vi "GoalKickKeeperTacticVSS.vi"(7 "First call?":bool=TRUE, 8 "error in (no error)":errorcluster, 9 "Game in":refnum<class "Game.lvclass">, 10 "Robot":refnum<class "Robot.lvclass">, 11 "GoalKickKeeperTacticVSS in":refnum<class "GoalKickKeeperTacticVSS.lvclass">) -> (0 "error out":errorcluster, 2 "Robot out":refnum<class "Robot.lvclass">, 3 "GoalKickKeeperTacticVSS out":refnum<class "GoalKickKeeperTacticVSS.lvclass">, 5 "x .or. y?":bool)   [LabVIEW 2020, in "GoalKickKeeperTacticVSS.lvclass"]
uses:
  GoalKickKeeperTacticVSS.lvclass
  C:/Users/pedro/Desktop/SSL_AI/Tactic_class/Tactic.lvclass
  Robot_class/Robot.lvclass
  Game_class/Game.lvclass
  Robot_class/tactics.ctl
  Tactic_class/Tactic.lvclass/Tactic.ctl
  Game_class/Game.lvclass/Game.ctl
  Robot_class/Robot.lvclass/Robot.ctl
  Game_class/Read BallRef.vi
  Tactic_class/Read Skillbook.vi
  Robot_class/Write tactic.vi
  Skillbook_class/Skillbook.lvclass
  KickSkillVSS_class/KickSkillVSS.lvclass
  PenaltyPosSkillVSS_class/PenaltyPosSkillVSS.lvclass
  BallDispPosSkillVSS_class/BallDispPosSkillVSS.lvclass
  BallToGoalSkillVSS_class/BallToGoalSkillVSS.lvclass
  GoToBallSkillVSS_class/GoToBallSkillVSS.lvclass
  DefBallPosSkillVSS_class/DefBallPosSkillVSS.lvclass
  HaltSkill_class/HaltSkill.lvclass
  KeeperDefPosSkillVSS_class/KeeperDefPosSkillVSS.lvclass
  GoToBallKeeperSkillVSS_class/GoToBallKeeperSkillVSS.lvclass
  Ball_class/Ball.lvclass
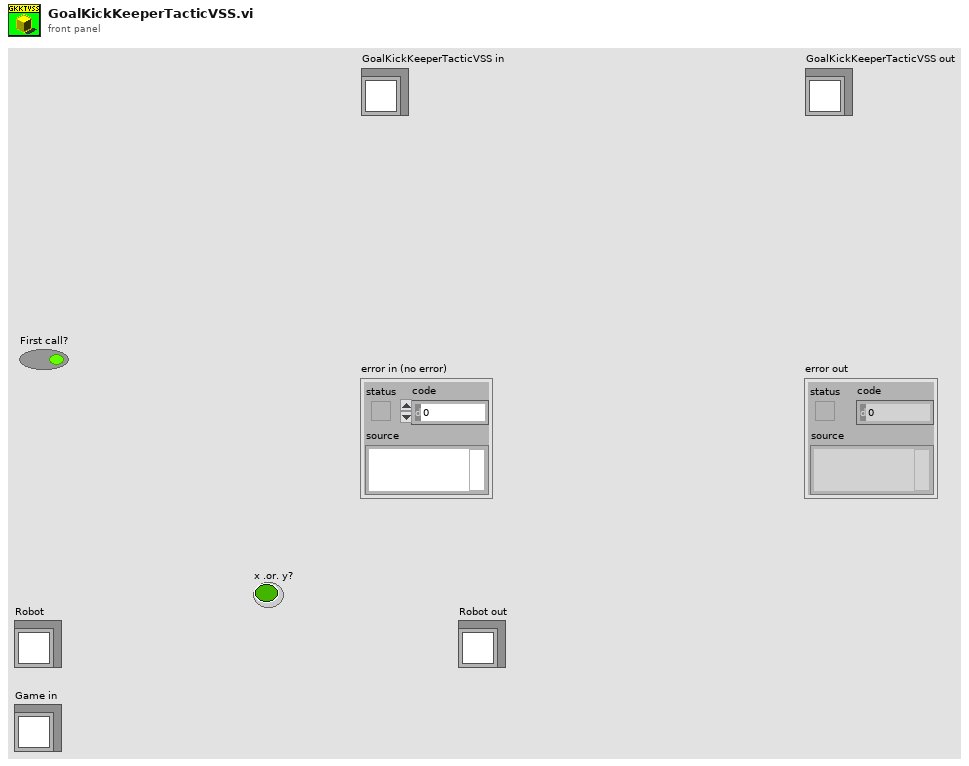
[diagram p1: front panel]
types:
  T1 = typedef "tactics.ctl" = enum16{"ReceivePassInFuturePoint", "Roller", "PrepareRollToPassRollerGoTo", "PrepareRollToPassReceiverGoTo", "WaitRoll", "PositionToRoll", "PenaltyAttacker", "PassObserver", "PenaltyDefense", "TableReceiverTactic", "Test", "DefendGoal", "Marker", "FollowAttacker", "DefendArea", "Shoot", "AttackerAimGoal", "AttackerBallOutOfField", "AttackerBlock", "AttackerStop", "Duelist", "Halt", "ZigZag", "GoTo", "Timeout", "KickToPassReceiver", "PositionToReceivePass", "DefendAreaVSS", "DefendGoalVSS", "KickVSS", "AttackVSS", "DispBallVSS", "PenaltyAttackVSS", "WaitPass"}
  T2 = cluster{"KickSkillVSS":refnum<class "KickSkillVSS.lvclass">, "PenaltyPosSkillVSS":refnum<class "PenaltyPosSkillVSS.lvclass">, "BallDispPosSkillVSS":refnum<class "BallDispPosSkillVSS.lvclass">, "BallToGoalSkillVSS":refnum<class "BallToGoalSkillVSS.lvclass">, "GoToBallSkillVSS":refnum<class "GoToBallSkillVSS.lvclass">, "DefBallPosSkillVSS":refnum<class "DefBallPosSkillVSS.lvclass">, "HaltSkill":refnum<class "HaltSkill.lvclass">, "KeeperDefPosSkillVSS":refnum<class "KeeperDefPosSkillVSS.lvclass">, "GoToBallKeeperSkillVSS":refnum<class "GoToBallKeeperSkillVSS.lvclass">}
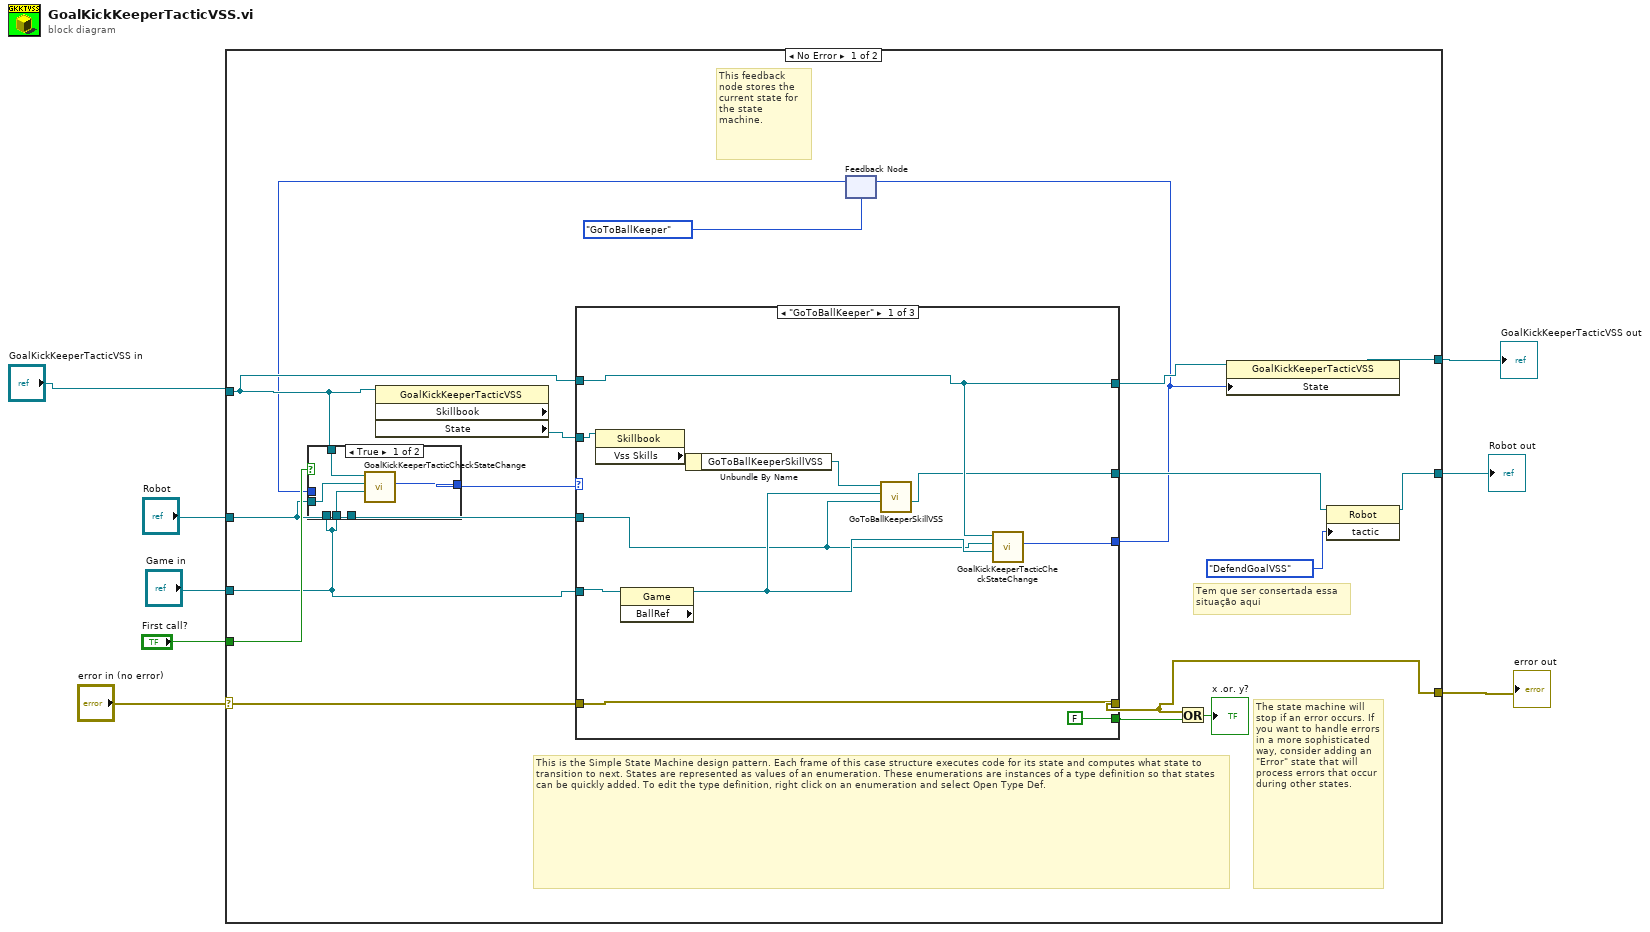
[diagram p0: block diagram]
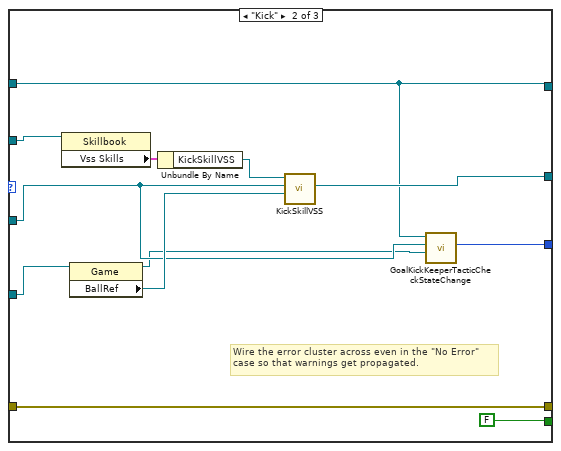
[diagram p2: hidden frame]
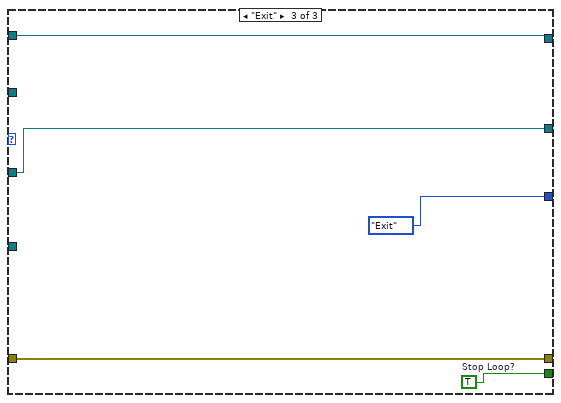
[diagram p3: hidden frame]
diagram:
  n1 = case shown="No Error" "error in (no error)" {
    selector: "error in (no error)" -> [w16 w62]
    tunnel: [w17 w62] -> w2
    tunnel: [w26 w61] -> w1
    tunnel: "GoalKickKeeperTacticVSS in" -> [w20 w61]
    tunnel: "Robot" -> [w12 w60]
    tunnel: "Game in" -> [w11 _]
    tunnel: [w24 w60] -> w5
    tunnel: "First call?" -> [w23 _]
    frame No Error {
      # "Tem que ser consertada essa \nsituação aqui"
      # "The state machine will stop if an error occurs. If you want to handle errors in a more sophisticated way, consider adding an \"Error\" state that will process errors that occur during other states."
      # "This feedback node stores the current state for the state machine."
      # "This is the Simple State Machine design pattern. Each frame of this case structure executes code for its state and computes what state to transition to next. States are represented as values of an enumeration. These enumerations are instances of a type definition so that states can be quickly added. To edit the type definition, right click on an enumeration and select Open Type Def."
      n2 = property class="GoalKickKeeperTacticVSS" props=["Skillbook", "State"](reference=w20) -> ("Skillbook"=w15:refnum<class "Skillbook.lvclass">)  [unwired: 1 in, 3 out]
      n3 = feedback #1(enum16{"GoToBallKeeper", "Kick", "Exit"}."GoToBallKeeper" ("State")) -> (w13:enum16{"GoToBallKeeper", "Kick", "Exit"})
      n4 = case shown="True" w23 {
        tunnel: w20 -> [w55 _]
        tunnel: w12 -> [_ _]
        tunnel: w11 -> [w58 _]
        tunnel: [w56 w59] -> w14
        tunnel: w13 -> [_ w59]
        tunnel: w12 -> [w57 _]
        tunnel: w11 -> [_ _]
        frame True {
          n5 = call "GoalKickKeeperTacticCheckStateChange.vi"("Game in"=w58, "Robot In"=w57, "GoalKickKeeperTacticVSS in"=w55) -> ("States"=w56:enum16{"GoToBallKeeper", "Kick", "Exit"})  [unwired: 6 in, 2 out]
        }
        frame False {
        }
      }
      n6 = case shown="\"GoToBallKeeper\"" w14 {
        tunnel: w11 -> [w36 w46 _]
        tunnel: w12 -> [w28 w40 w52]
        tunnel: [w27 w44 w52] -> w21
        tunnel: w20 -> [w31 w38 w51]
        tunnel: [w31 w38 w51] -> w19
        tunnel: [w32 w41 enum16{"GoToBallKeeper", "Kick", "Exit"}."Exit" ("State")] -> w9
        tunnel: [FALSE ("Stop Loop?") FALSE ("Stop Loop?") w53] -> w18
        tunnel: [w35 w43 w54] -> w17
        tunnel: w16 -> [w35 w43 w54]
        tunnel: w15 -> [w34 w47 _]
        frame "GoToBallKeeper" {
          n7 = property class="Skillbook"(reference=w34) -> ("Vss Skills"=w37:T2)  [unwired: 1 in, 2 out]
          n8 = property class="Game" props=["BallRef"](reference=w36) -> (reference out=w29:refnum<class "Game.lvclass">)  [unwired: 1 in, 2 out]
          n9 = Unbundle By Name(w37) -> ("GoToBallKeeperSkillVSS"=w30:refnum<class "GoToBallKeeperSkillVSS.lvclass">)
          n10 = call "GoToBallKeeperSkillVSS.vi"("Robot in"=w28, "Game in"=w29, "GoToBallKeeperSkillVSS in"=w30) -> ("Robot out"=w27:refnum<class "Robot.lvclass">)  [unwired: 6 in, 2 out]
          n11 = call "GoalKickKeeperTacticCheckStateChange.vi"("Game in"=w29, "Robot In"=w28, "GoalKickKeeperTacticVSS in"=w31) -> ("States"=w32:enum16{"GoToBallKeeper", "Kick", "Exit"})  [unwired: 6 in, 2 out]
        }
        frame "Kick" {
          # "Wire the error cluster across even in the \"No Error\"\ncase so that warnings get propagated."
          n12 = property class="Skillbook"(reference=w47) -> ("Vss Skills"=w49:T2)  [unwired: 1 in, 2 out]
          n13 = property class="Game"(reference=w46) -> (reference out=w39:refnum<class "Game.lvclass">, "BallRef"=w45:refnum<class "Ball.lvclass">)  [unwired: 1 in, 1 out]
          n14 = Unbundle By Name(w49) -> ("KickSkillVSS"=w48:refnum<class "KickSkillVSS.lvclass">)
          n15 = call-dynamic "KickSkillVSS.vi"("BallRef"=w45, "Robot"=w40, "KickSkillVSS in"=w48) -> ("Robot out"=w44:refnum<class "Robot.lvclass">)  [unwired: 6 in, 2 out]
          n16 = call "GoalKickKeeperTacticCheckStateChange.vi"("Game in"=w39, "Robot In"=w40, "GoalKickKeeperTacticVSS in"=w38) -> ("States"=w41:enum16{"GoToBallKeeper", "Kick", "Exit"})  [unwired: 6 in, 2 out]
        }
        frame "Exit" {
          w53 = TRUE  # Stop Loop?
        }
      }
      n17 = feedback-in #1(w9) -> ()
      n18 = Or(x=w17, y=w18) -> (x .or. y?=→"x .or. y?":bool)
      n19 = property class="GoalKickKeeperTacticVSS"(reference=w19, "State"=w9) -> (reference out=w26:refnum<class "GoalKickKeeperTacticVSS.lvclass">)  [unwired: 1 in, 1 out]
      n20 = property class="Robot"(reference=w21, "tactic"=tactics."DefendGoalVSS") -> (reference out=w24:refnum<class "Robot.lvclass">)  [unwired: 1 in, 1 out]
    }
    frame Error {
    }
  }
  "error out" <- w2
  "GoalKickKeeperTacticVSS out" <- w1
  "Robot out" <- w5
